vi "ryangosling.vi"(11 "CHASSIS":T6 {"vOmega" format="%10.3f"; "vY" format="%10.3f"; "vX" format="%10.3f"}) -> (1 "out WheelStates":T1[](array[typedef]) {"Angle"."SIN" format="%13.4f"; "Angle"."COS" format="%13.4f"; "Angle"."VALUE" format="%13.4f"}, 3 "out SWERVE_DRIVE_KINEMATICS":T3 {"SavedModuleStates"."Angle"."SIN" format="%13.4f"; "SavedModuleStates"."Angle"."COS" format="%13.4f"; "SavedModuleStates"."Angle"."VALUE" format="%13.4f"; "PrevCoR"."Y" format="%14.3f"; "PrevCoR"."X" format="%14.3f"; "Modules"."Y" format="%14.3f"; "Modules"."X" format="%14.3f"})   [LabVIEW 2023]
uses:
  <vilib>/Rock Robotics/WPI/ThirdParty/JAS_Junk/TrajLib/TypeDef/CHASSIS_SPEEDS.ctl
  <vilib>/Rock Robotics/WPI/ThirdParty/JAS_Junk/TrajLib/TypeDef/SWERVE_DRIVE_KINEMATICS.ctl
  <vilib>/Analysis/Matrix/Datatypes/RealMatrix.ctl
  <vilib>/Rock Robotics/WPI/ThirdParty/JAS_Junk/TrajLib/TypeDef/TRANSLATION2D.ctl
  <vilib>/Rock Robotics/WPI/ThirdParty/JAS_Junk/TrajLib/TypeDef/SWERVE_DRIVE_MODULE_STATE.ctl
  <vilib>/Rock Robotics/WPI/ThirdParty/JAS_Junk/TrajLib/TypeDef/ROTATION2D.ctl
  <vilib>/Rock Robotics/WPI/ThirdParty/REV Robotics/REVLib/Typedef/Spark MAX Control Type.ctl
  <vilib>/Rock Robotics/WPI/ThirdParty/JAS_Junk/TrajLib/Rotation2d_Minus.vi
  <vilib>/Rock Robotics/WPI/ThirdParty/JAS_Junk/TrajLib/Rotation2d_GetRadians.vi
  <vilib>/Rock Robotics/WPI/ThirdParty/JAS_Junk/TrajLib/SwerveModuleState_New.vi
  <vilib>/Rock Robotics/WPI/ThirdParty/JAS_Junk/TrajLib/Rotation2d_RotateBy.vi
  <vilib>/Rock Robotics/WPI/ThirdParty/JAS_Junk/TrajLib/Rotation2d_UnaryMinus.vi
  <vilib>/Rock Robotics/WPI/ThirdParty/JAS_Junk/TrajLib/Rotation2d_CreateXY.vi
  <vilib>/Rock Robotics/WPI/ThirdParty/JAS_Junk/TrajLib/Util_CalcDist.vi
  <vilib>/Rock Robotics/WPI/ThirdParty/JAS_Junk/TrajLib/Trajectory_Library.lvlib
  <vilib>/Analysis/Matrix/NI_Matrix.lvlib
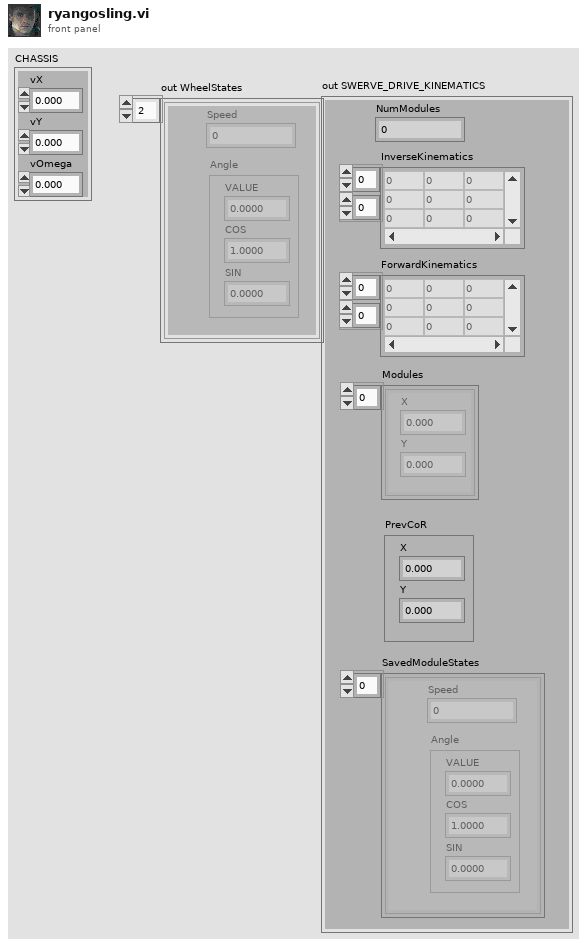
[diagram p1: front panel]
types:
  T1 = typedef "Trajectory_Library.lvlib/SWERVE_DRIVE_MODULE_STATE.ctl" = cluster{"Speed":dbl, "Angle":T2}
  T2 = typedef "Trajectory_Library.lvlib/ROTATION2D.ctl" = cluster{"VALUE":dbl, "COS":dbl, "SIN":dbl}
  T3 = typedef "Trajectory_Library.lvlib/SWERVE_DRIVE_KINEMATICS.ctl" = cluster{"NumModules":i32, "InverseKinematics":T4, "ForwardKinematics":T4, "Modules":T5[], "PrevCoR":T5, "SavedModuleStates":T1[]}
  T4 = typedef "NI_Matrix.lvlib/RealMatrix.ctl" = dbl[][]
  T5 = typedef "Trajectory_Library.lvlib/TRANSLATION2D.ctl" = cluster{"X":dbl, "Y":dbl}
  T6 = typedef "Trajectory_Library.lvlib/CHASSIS_SPEEDS.ctl" = cluster{"vX":dbl, "vY":dbl, "vOmega":dbl}
  T7 = typedef "Spark MAX Control Type.ctl" = enum16{"Percent VBus", "Voltage", "Velocity", "Position", "Smart Motion", "Current", "Smart Velocity"}
  T8 = typedef "WPI_MotorControlDeviceRef.ctl" = cluster{"DeviceStatus":errorcluster, "Type":T9, "PWM":cluster{"PWM Channel":T10, "DeadBand":T11}, "CAN":cluster{"Device Number":u8, "SetOutput VI Ref":variant, "GetOutput VI Ref":variant, "Enable VI Ref":variant, "Disable VI Ref":variant, "Data":variant}, "Invert":bool, "DIO PWM":cluster{"PWM \"Enable\" Channel":T10, "DIOChannel":T12, "PWM Rate":dbl}}
  T9 = typedef "WPI_MotorControlType.ctl" = enum16{"PWM", "CAN", "DIO PWM"}
  T10 = typedef "FPGA_DIOPWMChannel.ctl" = enum8{"PWM 0", "PWM 1", "PWM 2", "PWM 3", "PWM 4", "PWM 5", "PWM 6", "PWM 7", "PWM 8", "PWM 9", "PWM MXP 0", "PWM MXP 1", "PWM MXP 2", "PWM MXP 3", "PWM MXP 4", "PWM MXP 5", "PWM MXP 6", "PWM MXP 7", "PWM MXP 8", "PWM MXP 9", "Invalid"}
  T11 = typedef "WPI_PWMDeadband.ctl" = cluster{"Name":string, "maxPositivePwm":i32, "minPositivePwm":i32, "centerPwm":i32, "maxNegativePwm":i32, "minNegativePwm":i32, "angularRange":u16}
  T12 = typedef "FPGA_DIOChannel.ctl" = enum8{"DIO 0", "DIO 1", "DIO 2", "DIO 3", "DIO 4", "DIO 5", "DIO 6", "DIO 7", "DIO 8", "DIO 9", "DIO MXP 0", "DIO MXP 1", "DIO MXP 2", "DIO MXP 3", "DIO MXP 4", "DIO MXP 5", "DIO MXP 6", "DIO MXP 7", "DIO MXP 8", "DIO MXP 9", "DIO MXP 10", "DIO MXP 11", "DIO MXP 12", "DIO MXP 13", "DIO MXP 14", "DIO MXP 15", "SPI Port CS1", "SPI Port CS2", "SPI Port CS3", "SPI Port MISO", "SPI Port MOSI", "Invalid"}
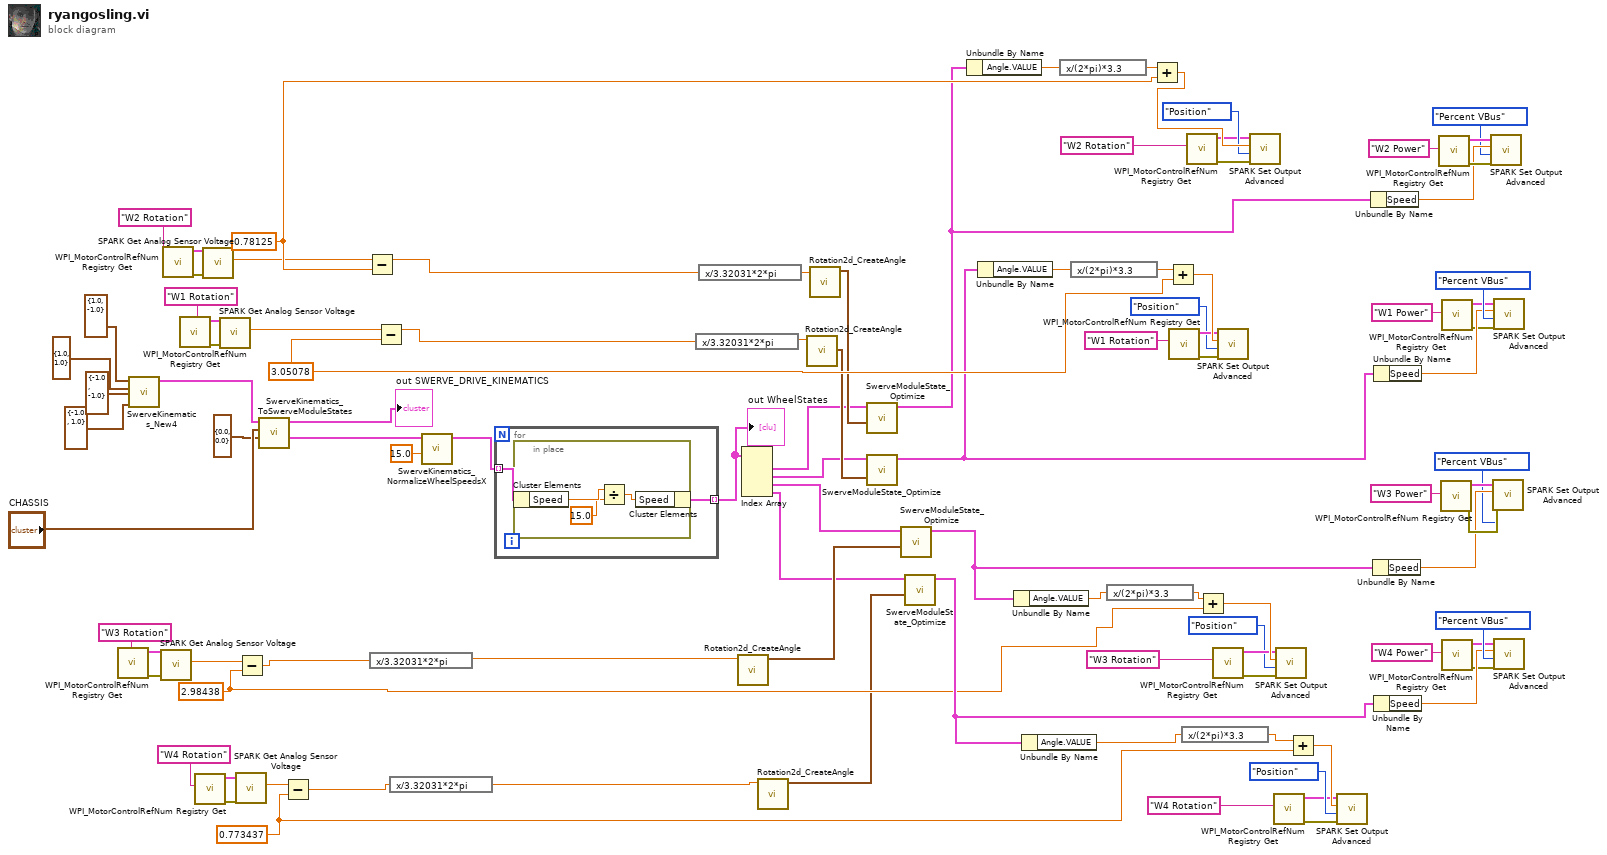
[diagram p0: block diagram]
diagram:
  w47 = 0.773437 ("x")
  w48 = 2.98438 ("y")
  w50 = 0.78125 ("y")
  w49 = 3.05078 ("y")
  n1 = call <vilib>:"WPI_MotorControlRefNum Registry Get.vi"("refnum name"="W3 Rotation") -> ("error out"=w18:errorcluster, "MotorControlDevRef"=w19:T8)  [unwired: 9 in]
  n2 = call <vilib>:"SwerveKinematics_New4.vi"("wheel 3"=T5 {"X"=-1.0, "Y"=1.0} ("wheel 0"), "wheel 2"=T5 {"X"=-1.0, "Y"=-1.0} ("wheel 0"), "wheel 1"=T5 {"X"=1.0, "Y"=1.0} ("wheel 0"), "wheel 0"=T5 {"X"=1.0, "Y"=-1.0}) -> ("SWERVE_DRIVE_KINEMATICS"=w10:T3)  [unwired: 7 in]
  n3 = call <vilib>:"SPARK Get Analog Sensor Voltage.vi"("error in (no error)"=w18, "MotorControlDevRef in"=w19) -> ("Analog Sensor Voltage"=w37:dbl)  [unwired: 6 in, 3 out]
  n4 = call <vilib>:"WPI_MotorControlRefNum Registry Get.vi"("refnum name"="W2 Rotation") -> ("error out"=w24:errorcluster, "MotorControlDevRef"=w25:T8)  [unwired: 9 in]
  n5 = call <vilib>:"WPI_MotorControlRefNum Registry Get.vi"("refnum name"="W1 Rotation") -> ("error out"=w27:errorcluster, "MotorControlDevRef"=w26:T8)  [unwired: 9 in]
  n6 = call <vilib>:"WPI_MotorControlRefNum Registry Get.vi"("refnum name"="W4 Rotation") -> ("error out"=w21:errorcluster, "MotorControlDevRef"=w20:T8)  [unwired: 9 in]
  n7 = call <vilib>:"SPARK Get Analog Sensor Voltage.vi"("error in (no error)"=w24, "MotorControlDevRef in"=w25) -> ("Analog Sensor Voltage"=w29:dbl)  [unwired: 6 in, 3 out]
  n8 = call <vilib>:"SPARK Get Analog Sensor Voltage.vi"("error in (no error)"=w27, "MotorControlDevRef in"=w26) -> ("Analog Sensor Voltage"=w32:dbl)  [unwired: 6 in, 3 out]
  n9 = call <vilib>:"SPARK Get Analog Sensor Voltage.vi"("error in (no error)"=w21, "MotorControlDevRef in"=w20) -> ("Analog Sensor Voltage"=w35:dbl)  [unwired: 6 in, 3 out]
  n10 = Subtract(x=w37, y=w48) -> (x-y=w45:dbl)
  n11 = call <vilib>:"SwerveKinematics_ToSwerveModuleStates.vi"("CenterOfRotation"=T5 {"X"=0.0, "Y"=0.0}, "ChassisSpeeds"="CHASSIS", "in SWERVE_DRIVE_KINEMATICS"=w10) -> ("ModuleStates"=w3:T1[], "out SWERVE_DRIVE_KINEMATICS"=→"out SWERVE_DRIVE_KINEMATICS":T3)  [unwired: 7 in]
  n12 = Subtract(x=w35, y=w47) -> (x-y=w46:dbl)
  n13 = Subtract(x=w29, y=w50) -> (x-y=w44:dbl)
  n14 = expression code="x/3.32031*2*pi"(w45) -> (w38:dbl)
  n15 = Subtract(x=w32, y=w49) -> (x-y=w43:dbl)
  n16 = expression code="x/3.32031*2*pi"(w46) -> (w36:dbl)
  n17 = call <vilib>:"SwerveKinematics_NormalizeWheelSpeedsX.vi"("AttainableMaxSpeed"=15.0, "in WheelStates"=w3) -> ("out WheelStates"=w2:T1[])  [unwired: 9 in]
  n18 = for {
    tunnel: w2 -> [w102] mode=indexing
    tunnel: [w101] -> w1 mode=indexing
    n19 = in-place {
      n20 = in-place-cluster #1(w102) -> ("Speed"=w104:dbl)
      n21 = Divide(x=w104, y=15.0) -> (x/y=w105:dbl)
      n22 = in-place-cluster #1("Speed"=w105) -> (w101:T1)
    }
  }
  "out WheelStates" <- w1
  n23 = expression code="x/3.32031*2*pi"(w43) -> (w33:dbl)
  n24 = expression code="x/3.32031*2*pi"(w44) -> (w30:dbl)
  n25 = call <vilib>:"Rotation2d_CreateAngle.vi"("Angle"=w38) -> ("ROTATION"=w39:T2)  [unwired: 10 in]
  n26 = Index Array(array=w1) -> (element #1=w13:T1, element #2=w16:T1, element #3=w15:T1, element #4=w14:T1)  [unwired: 4 in]
  n27 = call <vilib>:"Rotation2d_CreateAngle.vi"("Angle"=w36) -> ("ROTATION"=w40:T2)  [unwired: 10 in]
  n28 = call <vilib>:"Rotation2d_CreateAngle.vi"("Angle"=w33) -> ("ROTATION"=w34:T2)  [unwired: 10 in]
  n29 = call <vilib>:"Rotation2d_CreateAngle.vi"("Angle"=w30) -> ("ROTATION"=w31:T2)  [unwired: 10 in]
  n30 = call <vilib>:"SwerveModuleState_Optimize.vi"("CurrentAngle"=w31, "Desired State"=w13) -> ("out SWERVE_DRIVE_MODULE_STATE"=w41:T1)  [unwired: 9 in]
  n31 = call <vilib>:"SwerveModuleState_Optimize.vi"("CurrentAngle"=w34, "Desired State"=w16) -> ("out SWERVE_DRIVE_MODULE_STATE"=w42:T1)  [unwired: 9 in]
  n32 = call <vilib>:"SwerveModuleState_Optimize.vi"("CurrentAngle"=w39, "Desired State"=w15) -> ("out SWERVE_DRIVE_MODULE_STATE"=w86:T1)  [unwired: 9 in]
  n33 = call <vilib>:"SwerveModuleState_Optimize.vi"("CurrentAngle"=w40, "Desired State"=w14) -> ("out SWERVE_DRIVE_MODULE_STATE"=w87:T1)  [unwired: 9 in]
  n34 = Unbundle By Name(w41) -> ("Angle.VALUE"=w90:dbl)
  n35 = Unbundle By Name(w42) -> ("Angle.VALUE"=w92:dbl)
  n36 = Unbundle By Name(w86) -> ("Angle.VALUE"=w95:dbl)
  n37 = Unbundle By Name(w87) -> ("Angle.VALUE"=w100:dbl)
  n38 = expression code="x/(2*pi)*3.3"(w90) -> (w89:dbl)
  n39 = expression code="x/(2*pi)*3.3"(w92) -> (w93:dbl)
  n40 = expression code="x/(2*pi)*3.3"(w95) -> (w96:dbl)
  n41 = Add(x=w89, y=w50) -> (x+y=w91:dbl)
  n42 = Add(x=w93, y=w49) -> (x+y=w94:dbl)
  n43 = call <vilib>:"WPI_MotorControlRefNum Registry Get.vi"("refnum name"="W1 Rotation") -> ("error out"=w64:errorcluster, "MotorControlDevRef"=w63:T8)  [unwired: 9 in]
  n44 = expression code="x/(2*pi)*3.3"(w100) -> (w98:dbl)
  n45 = call <vilib>:"WPI_MotorControlRefNum Registry Get.vi"("refnum name"="W2 Rotation") -> ("error out"=w59:errorcluster, "MotorControlDevRef"=w60:T8)  [unwired: 9 in]
  n46 = Add(x=w96, y=w48) -> (x+y=w97:dbl)
  n47 = call <vilib>:"WPI_MotorControlRefNum Registry Get.vi"("refnum name"="W3 Rotation") -> ("error out"=w57:errorcluster, "MotorControlDevRef"=w56:T8)  [unwired: 9 in]
  n48 = call <vilib>:"SPARK Set Output Advanced.vi"("error in (no error)"=w64, "Control Mode"=Spark_MAX_Control_Type."Position", "Setpoint"=w94, "MotorControlDevRef"=w63) -> ()  [unwired: 6 in, 2 out]
  n49 = call <vilib>:"SPARK Set Output Advanced.vi"("error in (no error)"=w59, "Control Mode"=Spark_MAX_Control_Type."Position", "Setpoint"=w91, "MotorControlDevRef"=w60) -> ()  [unwired: 6 in, 2 out]
  n50 = call <vilib>:"WPI_MotorControlRefNum Registry Get.vi"("refnum name"="W4 Rotation") -> ("error out"=w52:errorcluster, "MotorControlDevRef"=w53:T8)  [unwired: 9 in]
  n51 = call <vilib>:"SPARK Set Output Advanced.vi"("error in (no error)"=w57, "Control Mode"=Spark_MAX_Control_Type."Position", "Setpoint"=w97, "MotorControlDevRef"=w56) -> ()  [unwired: 6 in, 2 out]
  n52 = Add(x=w98, y=w47) -> (x+y=w99:dbl)
  n53 = call <vilib>:"SPARK Set Output Advanced.vi"("error in (no error)"=w52, "Control Mode"=Spark_MAX_Control_Type."Position", "Setpoint"=w99, "MotorControlDevRef"=w53) -> ()  [unwired: 6 in, 2 out]
  n54 = Unbundle By Name(w41) -> ("Speed"=w68:dbl)
  n55 = Unbundle By Name(w86) -> ("Speed"=w78:dbl)
  n56 = Unbundle By Name(w42) -> ("Speed"=w73:dbl)
  n57 = Unbundle By Name(w87) -> ("Speed"=w83:dbl)
  n58 = call <vilib>:"WPI_MotorControlRefNum Registry Get.vi"("refnum name"="W2 Power") -> ("error out"=w70:errorcluster, "MotorControlDevRef"=w69:T8)  [unwired: 9 in]
  n59 = call <vilib>:"WPI_MotorControlRefNum Registry Get.vi"("refnum name"="W3 Power") -> ("error out"=w80:errorcluster, "MotorControlDevRef"=w79:T8)  [unwired: 9 in]
  n60 = call <vilib>:"WPI_MotorControlRefNum Registry Get.vi"("refnum name"="W1 Power") -> ("error out"=w71:errorcluster, "MotorControlDevRef"=w72:T8)  [unwired: 9 in]
  n61 = call <vilib>:"WPI_MotorControlRefNum Registry Get.vi"("refnum name"="W4 Power") -> ("error out"=w81:errorcluster, "MotorControlDevRef"=w82:T8)  [unwired: 9 in]
  n62 = call <vilib>:"SPARK Set Output Advanced.vi"("error in (no error)"=w70, "Control Mode"=Spark_MAX_Control_Type."Percent VBus", "Setpoint"=w68, "MotorControlDevRef"=w69) -> ()  [unwired: 6 in, 2 out]
  n63 = call <vilib>:"SPARK Set Output Advanced.vi"("error in (no error)"=w80, "Control Mode"=Spark_MAX_Control_Type."Percent VBus", "Setpoint"=w78, "MotorControlDevRef"=w79) -> ()  [unwired: 6 in, 2 out]
  n64 = call <vilib>:"SPARK Set Output Advanced.vi"("error in (no error)"=w71, "Control Mode"=Spark_MAX_Control_Type."Percent VBus", "Setpoint"=w73, "MotorControlDevRef"=w72) -> ()  [unwired: 6 in, 2 out]
  n65 = call <vilib>:"SPARK Set Output Advanced.vi"("error in (no error)"=w81, "Control Mode"=Spark_MAX_Control_Type."Percent VBus", "Setpoint"=w83, "MotorControlDevRef"=w82) -> ()  [unwired: 6 in, 2 out]
